vi "Array Add,Sub,Mult,Div.vi"() -> ()   [LabVIEW 2024]
panel:
  out "x/y":dbl[](array[numeric])
  out "x-y":dbl[](array[numeric])
  out "x*y":dbl[](array[numeric])
  out "x+y":dbl[](array[numeric])
  in  "Array 2":dbl[](array[numeric])
  in  "Array":dbl[](array[numeric])
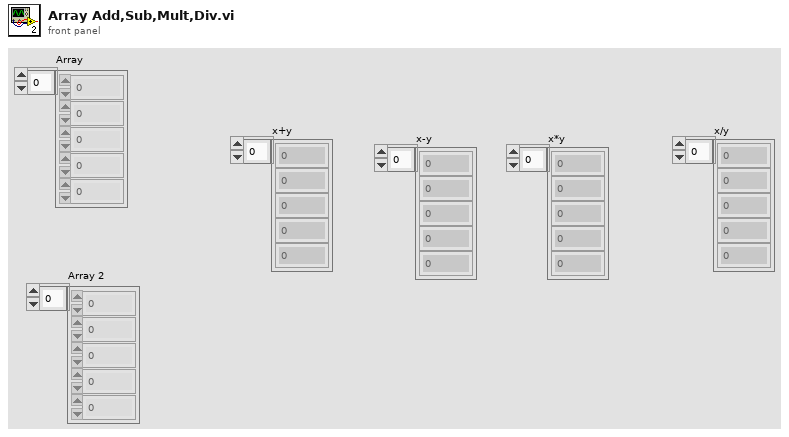
[diagram p1: front panel]
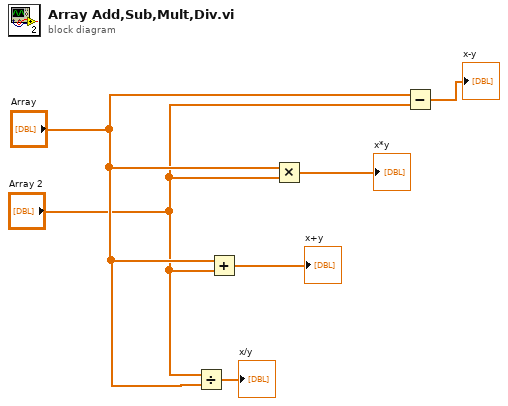
[diagram p0: block diagram]
diagram:
  n1 = Divide(x="Array 2", y="Array") -> (x/y=→"x/y":dbl[])
  n2 = Add(x="Array", y="Array 2") -> (x+y=→"x+y":dbl[])
  n3 = Multiply(x="Array", y="Array 2") -> (x*y=→"x*y":dbl[])
  n4 = Subtract(x="Array", y="Array 2") -> (x-y=→"x-y":dbl[])
